vi "Field Draw Target.vi"(4 "Lado":enum16{"Esquerdo", "Direito"}(ring) caption="Enum", 6 "Draw Targets?":T3, 7 "Robot":refnum<class "Robot.lvclass">, 8 "picture in":picture, 9 "Offset":T5, 10 "Scale mm/pixel":dbl, 11 "Project":T2=enum."VSS") -> (0 "picture out":picture)   [LabVIEW 2020]
uses:
  <vilib>/Utility/miscctls.llb/LVBoundsTypeDef.ctl
  <vilib>/Analysis/coordinate.llb/Angle Range (Degree).ctl
  DrawTargets.ctl
  Robot_class/Robot.lvclass
  Parameters_class/Project.ctl
  Robot_class/roles.ctl
  Robot_class/Robot.lvclass/Robot.ctl
  Controls/Functions Enum.ctl
  <vilib>/Analysis/coordinate.llb/2D Cartesian Coordinate Rotation (Scalar).vi
  Robot_class/Read dest_orientation.vi
  Robot_class/Read dest_x.vi
  Robot_class/Read dest_y.vi
  Robot_class/Read dest_x_kick.vi
  Robot_class/Read dest_y_kick.vi
  Robot_class/Read role.vi
  Robot_class/Read tactic.vi
  <vilib>/Analysis/NI_AAL_Angle.lvlib
  <vilib>/Analysis/NI_AALPro.lvlib
  <vilib>/Analysis/coordinate.llb/Wrap Angle (scalar).vi
panel:
  in  "RolesToDrawTargetKick":T1[](array[typedef])=[enum."PassBestRobot", enum."Shoot"]
  in  "angle range":T4=1
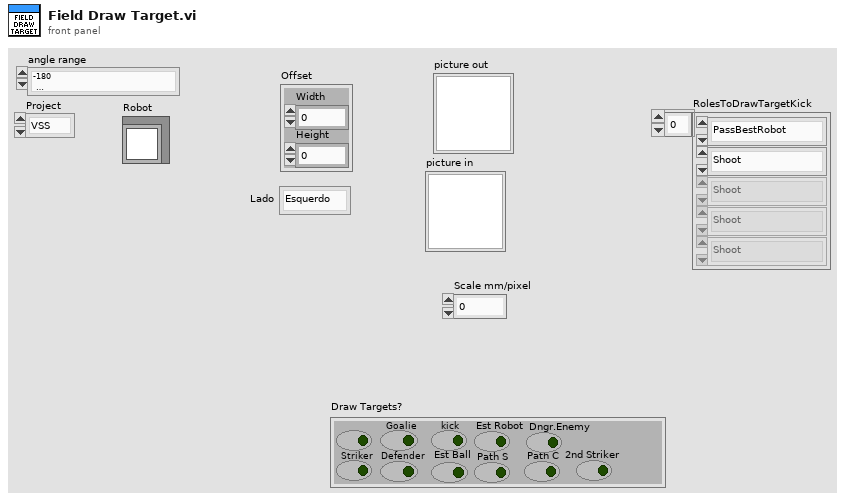
[diagram p1: front panel]
types:
  T1 = typedef "roles.ctl" = enum16{"SecondMarker", "5Robots5th", "PassBestReceiver", "5Robots4th", "5Robots3rd", "5Robots2nd", "5Robots1st", "PassBestRobot", "WaitPass", "ABCThirdKicker", "ABCFirstKicker", "ABCSecondKicker", "Tabler", "TableFinalizer", "PrepareRollToPassRoller", "PrepareRollToPassReceiver", "SimplePassRoll", "SimplePassRollReceiver", "PenaltyDefense", "PreparePassReceiver 2", "PreparePassReceiver 1", "PassObserver", "Timeout", "Goto", "ZigZag", "None", "BallOutOfField", "DefenderArea", "Duelist", "AttackerStop", "FollowAttacker", "KeeperRole", "KickPenalty", "AttackerAimGoal", "AttackerBlock", "Marker", "Halt", "Shoot", "PassKicker", "PassReceiver", "TestRole", "PenaltyAttacker"}
  T2 = typedef "Project.ctl" = enum16{"SSL", "VSS"}
  T3 = typedef "DrawTargets.ctl" = cluster{"Attacker":bool, "Striker":bool, "Goalie":bool, "Defender":bool, "kick":bool, "Est Ball":bool, "Est Robot":bool, "Path S":bool, "Path C":bool, "Dngr.Enemy":bool, "2nd Striker":bool}
  T4 = typedef "NI_AAL_Angle.lvlib/Angle Range (Degree).ctl" = u16
  T5 = typedef "LVBoundsTypeDef.ctl" = cluster{"Width":u32, "Height":u32}
  T6 = typedef "tactics.ctl" = enum16{"5Robots", "ReceivePassInFuturePoint", "Roller", "PrepareRollToPassRollerGoTo", "PrepareRollToPassReceiverGoTo", "WaitRoll", "PositionToRoll", "PenaltyAttacker", "PassObserver", "PenaltyDefense", "TableReceiverTactic", "Test", "DefendGoal", "Marker", "FollowAttacker", "DefendArea", "Shoot", "AttackerAimGoal", "AttackerBallOutOfField", "AttackerBlock", "AttackerStop", "Duelist", "Halt", "ZigZag", "GoTo", "Timeout", "KickToBestRobot", "KickToPassReceiver", "PositionToReceivePass", "WaitPass"}
  T7 = typedef "Functions Enum.ctl" = enum16{"2nd Striker", "Attacker", "Goalie", "Defender", "Striker", "Goto 0", "Dummy", "Kicker", "ZigZag 0", "ZigZag 1", "ZigZag 2", "ZigZag 3", "ZigZag 4", "ZigZag 5", "ZigZag 6", "ZigZag 7", "ZigZag 8", ""}
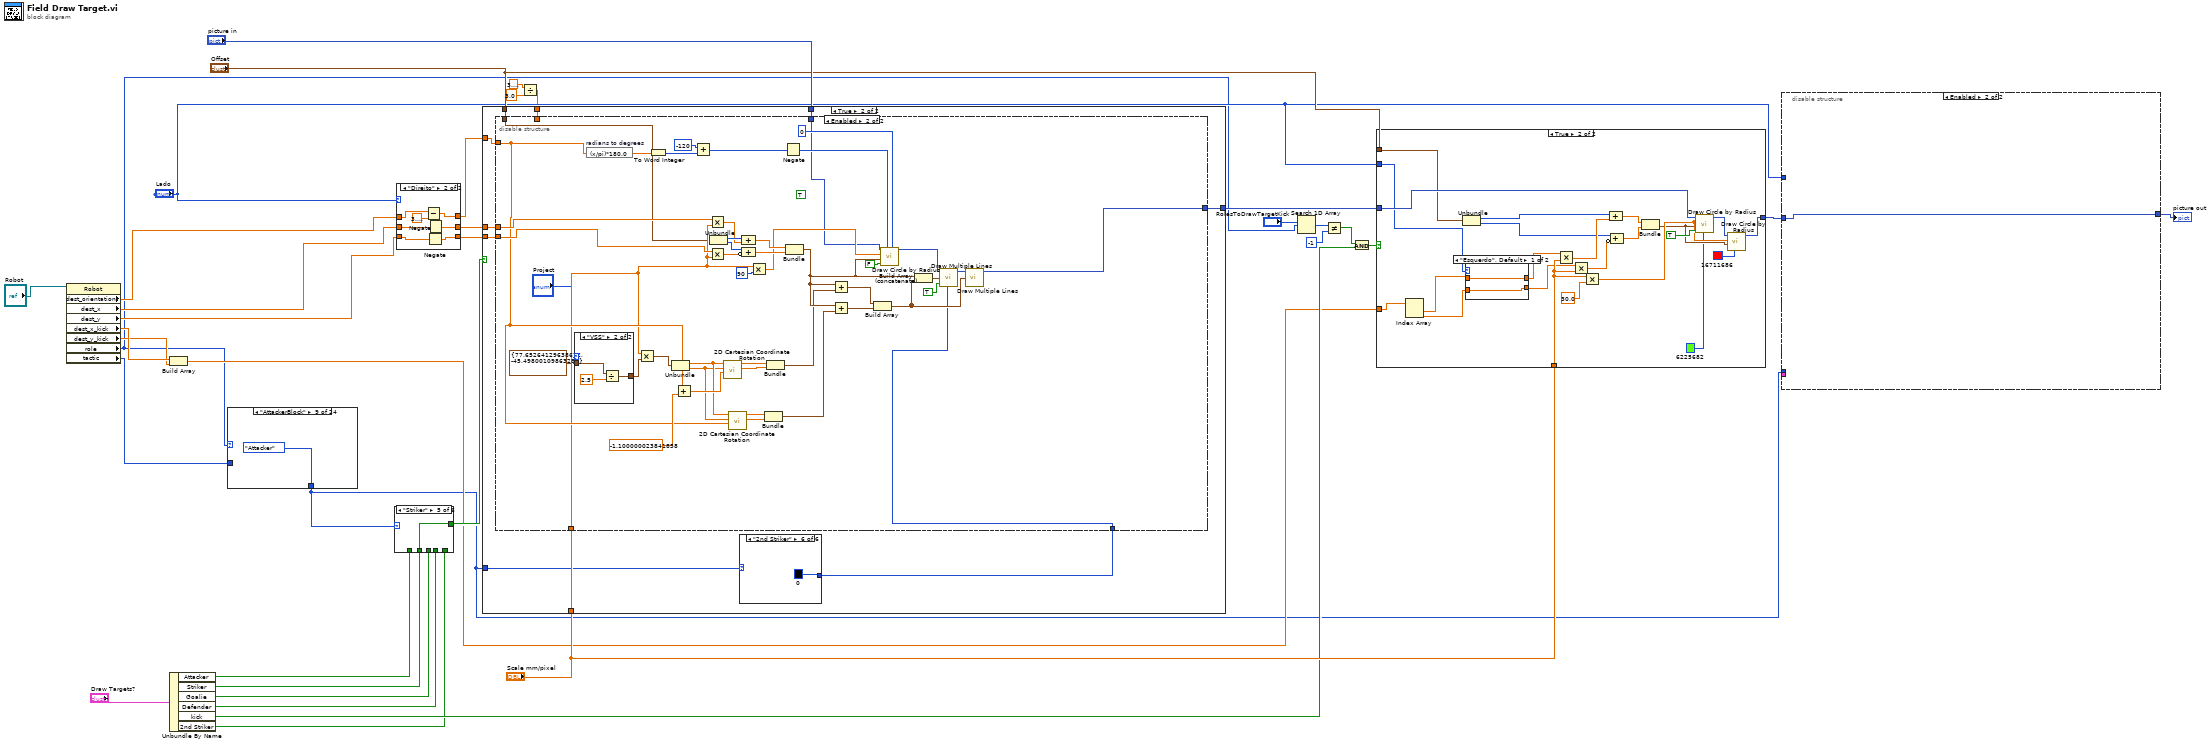
[diagram p0: block diagram]
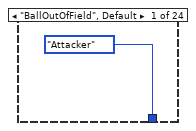
[diagram p2: hidden frame]
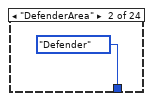
[diagram p3: hidden frame]
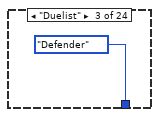
[diagram p4: hidden frame]
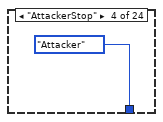
[diagram p5: hidden frame]
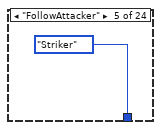
[diagram p6: hidden frame]
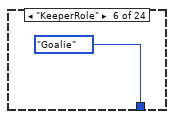
[diagram p7: hidden frame]
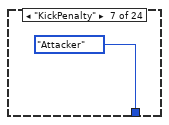
[diagram p8: hidden frame]
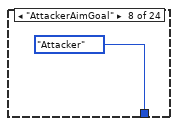
[diagram p9: hidden frame]
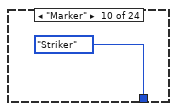
[diagram p10: hidden frame]
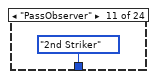
[diagram p11: hidden frame]
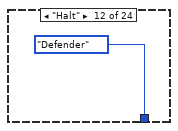
[diagram p12: hidden frame]
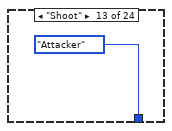
[diagram p13: hidden frame]
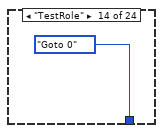
[diagram p14: hidden frame]
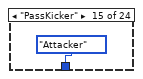
[diagram p15: hidden frame]
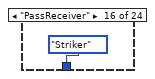
[diagram p16: hidden frame]
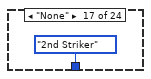
[diagram p17: hidden frame]
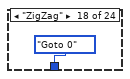
[diagram p18: hidden frame]
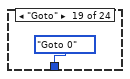
[diagram p19: hidden frame]
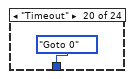
[diagram p20: hidden frame]
diagram:
  n1 = property class="Robot"(reference="Robot") -> ("dest_orientation"=w13:dbl, "dest_x"=w12:dbl, "dest_y"=w11:dbl, "dest_x_kick"=w10:dbl, "dest_y_kick"=w9:dbl, "role"=w4:T1, "tactic"=w6:T6)  [unwired: 1 in, 2 out]
  n2 = Unbundle By Name("Draw Targets?") -> ("Attacker"=w29:bool, "Striker"=w30:bool, "Goalie"=w28:bool, "Defender"=w31:bool, "kick"=w26:bool, "2nd Striker"=w15:bool)
  n3 = Build Array(w10, w9) -> (w8:dbl[])
  n4 = case shown="\"AttackerBlock\"" w4 {
    tunnel: [Functions_Enum."Attacker" ("function") Functions_Enum."Defender" ("function") Functions_Enum."Defender" ("function") Functions_Enum."Attacker" ("function") Functions_Enum."Striker" ("function") Functions_Enum."Goalie" ("function") Functions_Enum."Attacker" ("function") Functions_Enum."Attacker" ("function") Functions_Enum."Attacker" ("function") Functions_Enum."Striker" ("function") Functions_Enum."2nd Striker" ("function") Functions_Enum."Defender" ("function") Functions_Enum."Attacker" ("function") Functions_Enum."Goto 0" ("function") Functions_Enum."Attacker" ("function") Functions_Enum."Striker" ("function") Functions_Enum."2nd Striker" ("function") Functions_Enum."Goto 0" ("function") Functions_Enum."Goto 0" ("function") Functions_Enum."Goto 0" ("function") w58 Functions_Enum."2nd Striker" ("function") Functions_Enum."Attacker" ("function") Functions_Enum."Striker" ("function")] -> w7
    tunnel: w6 -> [_ _ _ _ _ _ _ _ _ _ _ _ _ _ _ _ _ _ _ _ w57 _ _ _]
    frame "BallOutOfField", Default {
    }
    frame "DefenderArea" {
    }
    frame "Duelist" {
    }
    frame "AttackerStop" {
    }
    frame "FollowAttacker" {
    }
    frame "KeeperRole" {
    }
    frame "KickPenalty" {
    }
    frame "AttackerAimGoal" {
    }
    frame "AttackerBlock" {
    }
    frame "Marker" {
    }
    frame "PassObserver" {
    }
    frame "Halt" {
    }
    frame "Shoot" {
    }
    frame "TestRole" {
    }
    frame "PassKicker" {
    }
    frame "PassReceiver" {
    }
    frame "None" {
    }
    frame "ZigZag" {
    }
    frame "Goto" {
    }
    frame "Timeout" {
    }
    frame "Tabler", "TableFinalizer" {
      n5 = case shown="\"Shoot\", \"KickToPassReceiver\"" w57 {
        tunnel: [Functions_Enum."Attacker" ("function") Functions_Enum."Striker" ("function")] -> w58
        frame "Shoot", "KickToPassReceiver" {
        }
        frame "WaitPass", Default {
        }
      }
    }
    frame "ABCThirdKicker" {
    }
    frame "ABCFirstKicker" {
    }
    frame "ABCSecondKicker" {
    }
  }
  n6 = case shown="\"Striker\"" w7 {
    tunnel: [w64 w65 TRUE ("Draw Target Striker?") w67 w68 w69] -> w32
    tunnel: w31 -> [_ _ _ w67 _ _]
    tunnel: w30 -> [_ _ _ _ w68 _]
    tunnel: w29 -> [w64 _ _ _ _ _]
    tunnel: w28 -> [_ w65 _ _ _ _]
    tunnel: w15 -> [_ _ _ _ _ w69]
    frame "Attacker", Default {
    }
    frame "Goalie" {
    }
    frame "Goto 0", "Kicker" {
    }
    frame "Defender" {
    }
    frame "Striker" {
    }
    frame "2nd Striker" {
    }
  }
  n7 = case shown="\"Direito\"" "Lado" {
    tunnel: [w72 w79] -> w25
    tunnel: w12 -> [w72 w76]
    tunnel: [w71 w77] -> w24
    tunnel: w11 -> [w71 w78]
    tunnel: w13 -> [w70 w74]
    tunnel: [w70 w75] -> w20
    frame "Esquerdo", Default {
    }
    frame "Direito" {
      n8 = Subtract(x=w74, y=3.141592653589793) -> (x-y=w75:dbl)
      n9 = Negate(x=w78) -> (-x=w77:dbl)
      n10 = Negate(x=w76) -> (-x=w79:dbl)
    }
  }
  n11 = Divide(x=3.141592653589793, y=3.0) -> (x/y=w19:dbl)
  n12 = case shown="True" w32 {
    tunnel: w24 -> [_ w89]
    tunnel: w25 -> [_ w88]
    tunnel: "picture in" -> [w80 w87]
    tunnel: [w80 w86] -> w35
    tunnel: "Offset" -> [_ w85]
    tunnel: "Scale mm/pixel" -> [_ w84]
    tunnel: w7 -> [_ w83]
    tunnel: w20 -> [_ w82]
    tunnel: w19 -> [_ w81]
    frame False {
    }
    frame True {
      n13 = case shown="\"2nd Striker\"" w83 {
        tunnel: [u32 14047743 ("color(black)") u32 16711680 ("color(black)") u32 11760127 ("color(black)") u32 4390883 ("color(black)") u32 16774186 ("color(black)") u32 0 ("color(black)")] -> w90
        frame "Goalie" {
        }
        frame "Attacker", Default {
        }
        frame "Goto 0", "Kicker" {
        }
        frame "Defender" {
        }
        frame "Striker" {
        }
        frame "2nd Striker" {
        }
      }
      n14 = disable-structure shown="Enabled" {
        disable-tunnel: w90 -> [w128 w134]
        disable-tunnel: w89 -> [w126 w139]
        disable-tunnel: w88 -> [w125 w140]
        disable-tunnel: w87 -> [w118 w137]
        disable-tunnel: [w114 w136] -> w86
        disable-tunnel: w85 -> [w113 w133]
        disable-tunnel: w84 -> [w112 w135]
        disable-tunnel: w82 -> [w103 w138]
        disable-tunnel: w81 -> [w100 _]
        frame Disabled {
          (unwired) 0.0 ("y")
          n15 = Unbundle(w113) -> ("Width"=w124:u32, "Height"=w121:u32)
          n16 = Divide(x=w100, y=2.0) -> (x/y=w102:dbl)
          n17 = Subtract(x=w103, y=w102) -> (x-y=w109:dbl)
          n18 = Multiply(x=w125, y=w112) -> (x*y=w123:dbl)
          n19 = Negate(x=w109) -> (-x=w108:dbl)
          n20 = Multiply(x=w126, y=w112) -> (x*y=w120:dbl)
          n21 = Divide(x=3.141592653589793, y=1.0) -> (x/y=w91:dbl)
          n22 = Multiply(x=w112, y=sgl 50.0 ("radius")) -> (x*y=w116:dbl)
          n23 = Subtract(x=w108, y=w91) -> (x-y=w104:dbl)
          n24 = Compound Arithmetic op=ADD(w124, w123) -> (w122:dbl)
          n25 = Compound Arithmetic op=ADD(w121, invert w120) -> (w119:dbl)
          n26 = call-poly <vilib>:"Wrap Angle.vi"("angle range"="angle range", "angle in"=w104) -> ("angle out"=w101:dbl)  [unwired: 8 in, 1 out]
          n27 = Bundle(w122, w119) -> (w115:cluster{dbl, dbl})  [unwired: 1 in]
          n28 = Multiply(x=w101, y=180.0) -> (x*y=w98:dbl)
          n29 = Divide(x=w98, y=3.141592653589793) -> (x/y=w93:dbl)
          n30 = Multiply(x=w100, y=180.0) -> (x*y=w99:dbl)
          n31 = Divide(x=w99, y=3.141592653589793) -> (x/y=w92:dbl)
          n32 = call <vilib>:"Draw Circle by Radius.vi"("arc size(360)"=w92, "color(black)"=w128, "start angle(0)"=w93, "fill?(F)"=TRUE, "pixel center"=w115, "radius"=w116, "picture"=w118) -> ("new picture"=w117:picture)  [unwired: 4 in]
          n33 = call <vilib>:"Draw Circle by Radius.vi"("arc size(360)"=w92, "color(black)"=u32 16777215, "start angle(0)"=w93, "pixel center"=w115, "radius"=w116, "picture"=w117) -> ("new picture"=w114:picture)  [unwired: 5 in]
        }
        frame Enabled {
          (unwired) TRUE ("fill?(F)")
          n34 = case shown="\"VSS\"" "Project" {
            tunnel: cluster{sgl, sgl} {77.65264, -45.498} ("appended array") -> [w175 w178]
            tunnel: [w175 w176] -> w131
            frame "SSL", Default {
            }
            frame "VSS" {
              n35 = Divide(x=w178, y=2.5) -> (x/y=w176:cluster{dbl, dbl})
            }
          }
          n36 = expression code="(x/pi)*180.0" "radians to degrees"(w138) -> (w166:dbl)
          n37 = Multiply(x=w135, y=w131) -> (x*y=w146:cluster{dbl, dbl})
          n38 = To Word Integer(number=w166) -> (16bit integer=w165:i16)
          n39 = Unbundle(w146) -> (w150:dbl, w149:dbl)
          n40 = Add(x=w138, y=sgl -1.1 ("theta")) -> (x+y=w151:dbl)
          n41 = Add(x=i16 -120, y=w165) -> (x+y=w164:i16)
          n42 = Multiply(x=w140, y=w135) -> (x*y=w172:dbl)
          n43 = Multiply(x=w139, y=w135) -> (x*y=w169:dbl)
          n44 = Unbundle(w133) -> ("Width"=w173:u32, "Height"=w170:u32)
          n45 = call-poly <vilib>:"2D Cartesian Coordinate Rotation.vi"("theta"=w151, "y"=w149, "x"=w150) -> ("y out"=w153:dbl, "x out"=w154:dbl)  [unwired: 6 in, 1 out]
          n46 = call-poly <vilib>:"2D Cartesian Coordinate Rotation.vi"("theta"=w138, "y"=w149, "x"=w150) -> ("y out"=w147:dbl, "x out"=w148:dbl)  [unwired: 6 in, 1 out]
          n47 = Compound Arithmetic op=ADD(w173, w172) -> (w171:dbl)
          n48 = Compound Arithmetic op=ADD(w170, invert w169) -> (w168:dbl)
          n49 = Multiply(x=w135, y=i16 90 ("radius")) -> (x*y=w160:dbl)
          n50 = Bundle("x out"=w148, "y out"=w147) -> (w145:cluster{"x out":dbl, "y out":dbl})  [unwired: 1 in]
          n51 = Bundle("x out"=w154, "y out"=w153) -> (w144:cluster{"x out":dbl, "y out":dbl})  [unwired: 1 in]
          n52 = Negate(x=w164) -> (-x=w162:i16)
          n53 = Bundle(w171, w168) -> (w159:cluster{dbl, dbl})  [unwired: 1 in]
          n54 = Add(x=w159, y=w144) -> (x+y=w142:cluster{dbl, dbl})
          n55 = Add(x=w159, y=w145) -> (x+y=w143:cluster{dbl, dbl})
          n56 = Build Array(w142, w143) -> (w158:cluster{dbl, dbl}[])
          n57 = call <vilib>:"Draw Circle by Radius.vi"("arc size(360)"=i16 0, "start angle(0)"=w162, "fill?(F)"=FALSE, "pixel center"=w159, "radius"=w160, "picture"=w137) -> ("new picture"=w141:picture)  [unwired: 5 in]
          n58 = Build Array (concatenate)(w159, w158) -> (w156:cluster{dbl, dbl}[])
          n59 = call <vilib>:"Draw Multiple Lines.vi"("picture"=w141, "line endpoints"=w156, "fill?(F)"=TRUE, "color(black)"=w134) -> ("new picture"=w157:picture)  [unwired: 5 in]
          n60 = call <vilib>:"Draw Multiple Lines.vi"("picture"=w157, "line endpoints"=w158) -> ("new picture"=w136:picture)  [unwired: 7 in]
        }
      }
    }
  }
  n61 = Search 1D Array(1D array="RolesToDrawTargetKick", element=w4) -> (index of element=w3:i32)  [unwired: 1 in]
  n62 = Not Equal?(x=w3, y=-1) -> (x != y?=w1:bool)
  n63 = And(x=w1, y=w26) -> (x .and. y?=w27:bool)
  n64 = case shown="True" w27 {
    tunnel: w35 -> [w185 w197]
    tunnel: [w185 w196] -> w23
    tunnel: "Offset" -> [_ w195]
    tunnel: "Scale mm/pixel" -> [_ w194]
    tunnel: "Lado" -> [_ w189]
    tunnel: w8 -> [_ w188]
    frame False {
    }
    frame True {
      n65 = Index Array(array=w188) -> (element #1=w187:dbl, element #2=w186:dbl)  [unwired: 2 in]
      n66 = Unbundle(w195) -> ("Width"=w206:u32, "Height"=w203:u32)
      n67 = case shown="\"Esquerdo\", Default" w189 {
        tunnel: [w210 w214] -> w191
        tunnel: w187 -> [w210 w212]
        tunnel: [w209 w213] -> w190
        tunnel: w186 -> [w209 w211]
        frame "Esquerdo", Default {
        }
        frame "Direito" {
          n68 = Negate(x=w211) -> (-x=w213:dbl)
          n69 = Negate(x=w212) -> (-x=w214:dbl)
        }
      }
      n70 = Multiply(x=w191, y=w194) -> (x*y=w205:dbl)
      n71 = Multiply(x=w190, y=w194) -> (x*y=w202:dbl)
      n72 = Multiply(x=w194, y=sgl 30.0 ("radius")) -> (x*y=w199:dbl)
      n73 = Compound Arithmetic op=ADD(w206, w205) -> (w204:dbl)
      n74 = Compound Arithmetic op=ADD(w203, invert w202) -> (w201:dbl)
      n75 = Bundle(w204, w201) -> (w198:cluster{dbl, dbl})  [unwired: 1 in]
      n76 = call <vilib>:"Draw Circle by Radius.vi"("color(black)"=u32 6225682, "fill?(F)"=TRUE, "pixel center"=w198, "radius"=w199, "picture"=w197) -> ("new picture"=w200:picture)  [unwired: 6 in]
      n77 = call <vilib>:"Draw Circle by Radius.vi"("color(black)"=u32 16711686, "pixel center"=w198, "radius"=w199, "picture"=w200) -> ("new picture"=w196:picture)  [unwired: 7 in]
    }
  }
  n78 = disable-structure shown="Enabled" {
    disable-tunnel: w23 -> [w224 w244]
    disable-tunnel: w7 -> [w223 _]
    disable-tunnel: [w217 w244] -> w22
    disable-tunnel: _ -> [w216 _]
    disable-tunnel: "Lado" -> [w215 _]
    frame Disabled {
      n79 = Equal?(x=Functions_Enum."Striker", y=w223) -> (x = y?=w218:bool)
      n80 = Equal?(x=Functions_Enum."Attacker", y=w223) -> (x = y?=w219:bool)
      n81 = Or(x=w219, y=w218) -> (x .or. y?=w220:bool)
      n82 = case shown="True" w220 {
        tunnel: w224 -> [w225 w233]
        tunnel: [w225 w234] -> w217
        tunnel: w216 -> [_ w237]
        tunnel: w215 -> [_ w227]
        frame False {
        }
        frame True {
          n83 = Unbundle By Name(w237) -> ("Gap Coord"=w235)
          n84 = Index Array(array=w235) -> (element #1=w230, element #2=w229)  [unwired: 2 in]
          n85 = case shown="\"Esquerdo\", Default" w227 {
            tunnel: [w239 w243] -> _
            tunnel: w230 -> [w239 w241]
            tunnel: [w238 w242] -> w228
            tunnel: w229 -> [w238 w240]
            frame "Esquerdo", Default {
            }
            frame "Direito" {
              n86 = Negate(x=w240) -> (-x=w242:dbl)
              n87 = Negate(x=w241) -> (-x=w243:dbl)
            }
          }
          n88 = Bundle By Name(cluster=cluster{"x":i16, "y":i16} {"x"=0, "y"=0} ("end point"), "x"=i16 -4500, "y"=w228) -> (w232:cluster{"x":i16, "y":i16})
          n89 = call <vilib>:"Draw Line.vi"("picture"=w233, "end point"=w232, "color(black)"=u32 6618880) -> ("new picture"=w234:picture)  [unwired: 6 in]
        }
      }
    }
    frame Enabled {
    }
  }
  "picture out" <- w22
